vi "Event Log - Start.vi"() -> ()   [LabVIEW 2011]
uses:
  Event Log - Priority.ctl
panel:
  out "VI Started":string
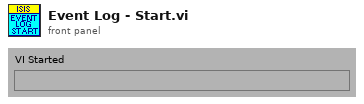
[diagram p1: front panel]
types:
  T1 = typedef "Event Log - Priority.ctl" = enum16{"None", "Log", "SECI and Log"}
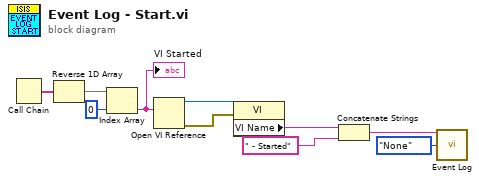
[diagram p0: block diagram]
diagram:
  n1 = Call Chain() -> (call chain=w9:string[])
  n2 = Reverse 1D Array(array=w9) -> (reversed array=w8:string[])
  n3 = Index Array(array=w8, index=0) -> (element=w1:string)
  "VI Started" <- w1
  n4 = Open VI Reference(vi path=w1) -> (vi reference=w6:refnum<vi>, error out=w5:errorcluster)  [unwired: 5 in]
  n5 = property class="VI"(reference=w6, error in=w5) -> ("VI Name"=w4:string)  [unwired: 2 out]
  n6 = Concatenate Strings(w4, " - Started") -> (w2:string)
  n7 = call "Event Log.vi"("Event log message"=w2, "Priority"=Event_Log_-_Priority."None") -> ()  [unwired: 13 in, 1 out]
